vi "DAQ_zero_ALL.vi"(1 "error in":errorcluster) -> (0 "error out":errorcluster)   [LabVIEW 2015]
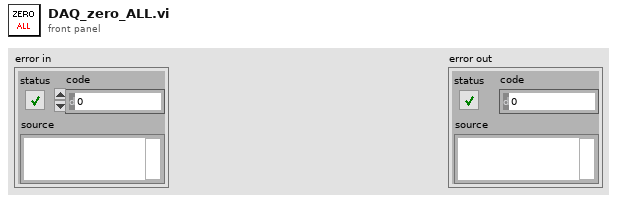
[diagram p1: front panel]
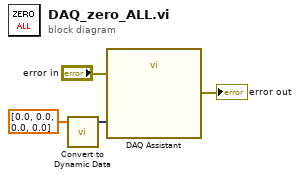
[diagram p0: block diagram]
diagram:
  n1 = call "Convert to Dynamic Data"("Array"=dbl[] [0.0, 0.0, 0.0, 0.0]) -> ("Dynamic Data Type"=w4:dynamicdata)  [unwired: 3 in]
  n2 = call "DAQ Assistant"("data"=w4, "error in"="error in") -> ("error out"=→"error out":errorcluster)  [unwired: 16 in, 1 out]
